vi "Run Test.vi"(8 "error in (no error)":errorcluster, 11 "Test Template in":refnum<class "Program Driver.lvclass">) -> (0 "error out":errorcluster, 1 "Positions":i32[](array[numeric]), 2 "Tests Passed":bool[](array[boolean]), 3 "Test Template out":refnum<class "Program Driver.lvclass">, 5 "Fail Codes":string[](array[string]))   [LabVIEW 2015, in "Program Driver.lvclass"]
uses:
  Program Driver.lvclass
  Test Class/Test Class.lvclass
  Classes/Application/Class/Application.lvclass
  Driver Test/Driver Test.lvclass
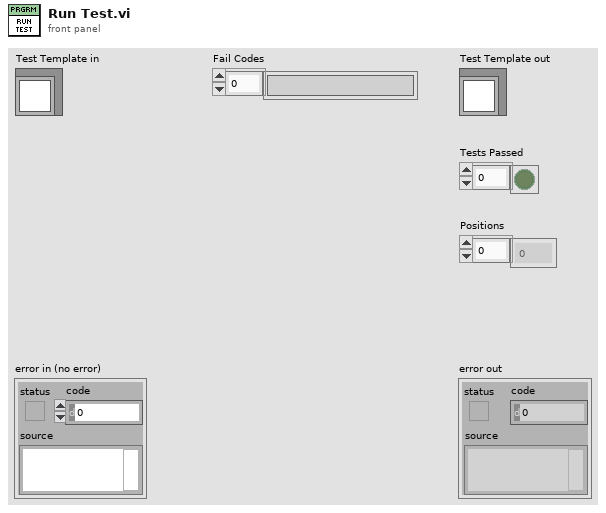
[diagram p1: front panel]
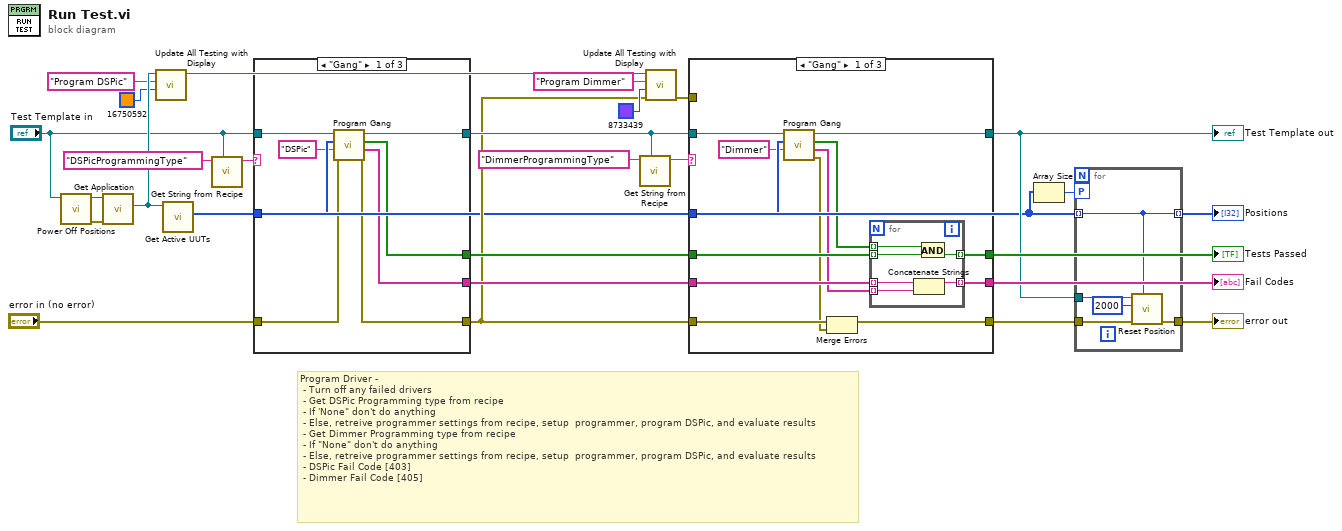
[diagram p0: block diagram]
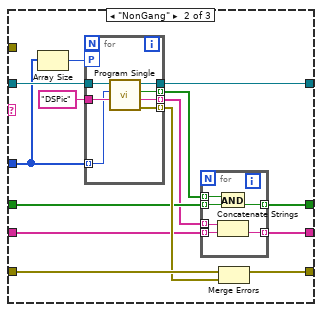
[diagram p2: hidden frame]
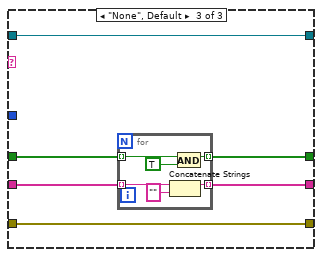
[diagram p3: hidden frame]
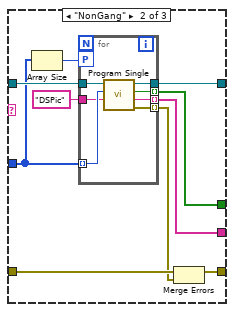
[diagram p4: hidden frame]
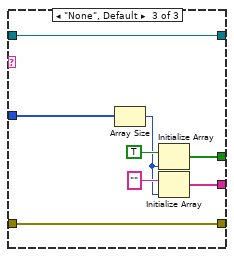
[diagram p5: hidden frame]
diagram:
  # "Program Driver -\n\t- Turn off any failed drivers\n\t- Get DSPic Programming type from recipe\n\t- If 'None\" don't do anything\n\t- Else, retreive programmer settings from recipe, setup \tprogrammer, program DSPic, and evaluate results\n\t- Get Dimmer Programming type from recipe\n\t- If \"None\" don't do anything\n\t- Else, retreive programmer settings from recipe, setup \tprogrammer, program DSPic, and evaluate results\n\t- DSPic Fail Code [403]\n\t- Dimmer Fail Code [405]"
  n1 = call "Power Off Positions.vi"("Driver Test"="Test Template in") -> ("error out"=w14:errorcluster)  [unwired: 10 in]
  n2 = call "Get Application.vi"("error in (no error)"=w14, "Test Class in"="Test Template in") -> ("Application.lvlib:Application.lvclass"=w25:refnum<class "Application.lvclass">)  [unwired: 8 in, 1 out]
  n3 = call "Update All Testing with Display.vi"("BG Color"=u32 16750592, "Message ('')"="Program DSPic", "Application in"=w25) -> ("Application out"=w9:refnum<class "Application.lvclass">)  [unwired: 7 in, 1 out]
  n4 = call "Get Active UUTs.vi"("Application in"=w25) -> ("Active Positions"=w2:u32[])  [unwired: 8 in, 2 out]
  n5 = call "Get String from Recipe.vi"("Test Class in"="Test Template in", "Name"="DSPicProgrammingType") -> ("Value"=w19:string)  [unwired: 7 in, 2 out]
  n6 = case shown="\"Gang\"" w19 {
    tunnel: "Test Template in" -> [w34 w44 w59]
    tunnel: [w33 w43 w59] -> w17
    tunnel: "error in (no error)" -> [w29 w37 w58]
    tunnel: [w28 w38 w58] -> w7
    tunnel: [w32 w39 w55] -> w15
    tunnel: [w31 w40 w54] -> w16
    tunnel: w2 -> [w30 w41 w56]
    frame "Gang" {
      n7 = call "Program Gang.vi"("error in (no error)"=w29, "Micro"="DSPic", "Active Positions"=w30, "Program Driver in"=w34) -> ("error out"=w28:errorcluster, "Fail Codes"=w31:string[], "Tests Passed"=w32:bool[], "Program Driver out"=w33:refnum<class "Program Driver.lvclass">)  [unwired: 4 in]
    }
    frame "NonGang" {
      n8 = Array Size(array=w41) -> (size(s)=w42:i32)
      n9 = for {
        tunnel: w41 -> [w49] mode=indexing
        workers-P: w42 -> [_]
        tunnel: [w48] -> w40 mode=indexing
        tunnel: [w47] -> w39 mode=indexing
        tunnel: [w46] -> w36 mode=indexing
        tunnel: "DSPic" ("Micro") -> [w45]
        tunnel: w44 -> [w51]
        tunnel: [w50] -> w43
        n10 = call "Program Single.vi"("Micro"=w45, "Positions"=w49, "Program Driver in"=w51) -> ("error out"=w46:errorcluster, "Fail Codes"=w48:string, "Tests Passed"=w47:bool, "Program Driver out"=w50:refnum<class "Program Driver.lvclass">)  [unwired: 5 in]
      }
      n11 = Merge Errors(w37, w36) -> (w38:errorcluster)
    }
    frame "None", Default {
      n12 = Array Size(array=w56) -> (size(s)=w52:i32)
      n13 = Initialize Array(TRUE ("Boolean"), w52) -> (w55:bool[])
      n14 = Initialize Array("" ("String"), w52) -> (w54:string[])
    }
  }
  n15 = call "Get String from Recipe.vi"("Test Class in"=w17, "Name"="DimmerProgrammingType") -> ("Value"=w18:string)  [unwired: 7 in, 2 out]
  n16 = call "Update All Testing with Display.vi"("error in (no error)"=w7, "BG Color"=u32 8733439, "Message ('')"="Program Dimmer", "Application in"=w9) -> ("error out"=w8:errorcluster)  [unwired: 6 in, 1 out]
  n17 = case shown="\"Gang\"" w18 {
    tunnel: w17 -> [w67 w87 w111]
    tunnel: [w66 w85 w111] -> w3
    tunnel: w7 -> [w65 w92 w110]
    tunnel: [w64 w84 w110] -> w6
    tunnel: w16 -> [w71 w81 w107]
    tunnel: w15 -> [w72 w82 w109]
    tunnel: [w70 w91 w108] -> w12
    tunnel: [w69 w90 w106] -> w13
    tunnel: w2 -> [w68 w86 _]
    tunnel: w8 -> [_ _ _]
    frame "Gang" {
      n18 = call "Program Gang.vi"("Micro"="Dimmer", "Active Positions"=w68, "Program Driver in"=w67) -> ("error out"=w63:errorcluster, "Fail Codes"=w62:string[], "Tests Passed"=w61:bool[], "Program Driver out"=w66:refnum<class "Program Driver.lvclass">)  [unwired: 5 in]
      n19 = Merge Errors(w65, w63) -> (w64:errorcluster)
      n20 = for {
        tunnel: w72 -> [w74] mode=indexing
        tunnel: [w78] -> w70 mode=indexing
        tunnel: w71 -> [w77] mode=indexing
        tunnel: [w76] -> w69 mode=indexing
        tunnel: w62 -> [w75] mode=indexing
        tunnel: w61 -> [w73] mode=indexing
        n21 = Concatenate Strings(w77, w75) -> (w76:string)
        n22 = And(x=w73, y=w74) -> (x .and. y?=w78:bool)
      }
    }
    frame "NonGang" {
      n23 = Array Size(array=w86) -> (size(s)=w88:i32)
      n24 = for {
        tunnel: w86 -> [w93] mode=indexing
        workers-P: w88 -> [_]
        tunnel: [w97] -> w80 mode=indexing
        tunnel: [w96] -> w79 mode=indexing
        tunnel: [w95] -> w83 mode=indexing
        tunnel: "DSPic" ("Micro") -> [w94]
        tunnel: w87 -> [w99]
        tunnel: [w98] -> w85
        n25 = call "Program Single.vi"("Micro"=w94, "Positions"=w93, "Program Driver in"=w99) -> ("error out"=w95:errorcluster, "Fail Codes"=w97:string, "Tests Passed"=w96:bool, "Program Driver out"=w98:refnum<class "Program Driver.lvclass">)  [unwired: 5 in]
      }
      n26 = for {
        tunnel: w82 -> [w102] mode=indexing
        tunnel: [w105] -> w91 mode=indexing
        tunnel: w81 -> [w104] mode=indexing
        tunnel: [w103] -> w90 mode=indexing
        tunnel: w80 -> [w100] mode=indexing
        tunnel: w79 -> [w101] mode=indexing
        n27 = And(x=w101, y=w102) -> (x .and. y?=w105:bool)
        n28 = Concatenate Strings(w100, w104) -> (w103:string)
      }
      n29 = Merge Errors(w92, w83) -> (w84:errorcluster)
    }
    frame "None", Default {
      n30 = for {
        tunnel: w109 -> [w117] mode=indexing
        tunnel: [w115] -> w108 mode=indexing
        tunnel: w107 -> [w114] mode=indexing
        tunnel: [w113] -> w106 mode=indexing
        n31 = Concatenate Strings(w114, "" ("string")) -> (w113:string)
        n32 = And(x=w117, y=TRUE) -> (x .and. y?=w115:bool)
      }
    }
  }
  "Test Template out" <- w3
  "Tests Passed" <- w12
  "Fail Codes" <- w13
  n33 = Array Size(array=w2) -> (size(s)=w1:i32)
  n34 = for {
    tunnel: w3 -> [w120]
    tunnel: w2 -> [w119] mode=indexing
    tunnel: [w119] -> w4 mode=indexing
    workers-P: w1 -> [_]
    tunnel: w6 -> [w122]
    tunnel: [w121] -> w5
    n35 = call "Reset Position.vi"("Position"=w119, "error in (no error)"=w122, "Wait After Power Off (1500 ms)"=u32 2000, "Driver Test"=w120) -> ("error out"=w121:errorcluster)  [unwired: 7 in]
  }
  "error out" <- w5
  "Positions" <- w4
